vi "Intake Set Modes.vi"   [LabVIEW 2016]
uses:
  Intake Control Type.ctl
  <vilib>/Rock Robotics/WPI/DriverStation/WPI_DriverStationRobotMode2.ctl
  Intake Globals.vi
  Robot Global Data.vi
types:
  T1 = typedef "WPI_DriverStationRobotMode2.ctl" = enum16{"Autonomous Disabled", "Autonomous Enabled", "Teleop Disabled", "Teleop Enabled", "Disconnected", "Finish", "Test Disabled", "Test Enabled", "Emergency Stopped"}
  T2 = typedef "Intake Control Type.ctl" = enum16{"No Op", "In", "Out"}
  T3 = typedef "Intake Notifier.ctl" = cluster{"In":bool, "Out":bool, "Intake Control List":T2, "Parameter 1":dbl, "Parameter 2":dbl, "Intake Notifier":refnum<notifier>, "Step":i32}
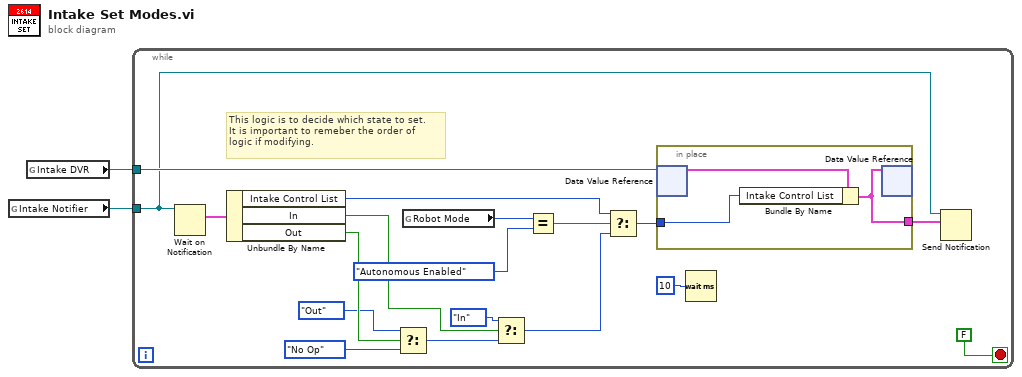
[diagram p0: block diagram]
diagram:
  n1 = global read "Intake Globals.vi" "Intake Notifier"() -> (w1:refnum<notifier>)
  n2 = global read "Intake Globals.vi" "Intake DVR"() -> (w2:refnum<data-value>)
  n3 = while {
    tunnel: w2 -> [w13]
    tunnel: w1 -> [w3]
    stop <- FALSE stop-if-true
    # "This logic is to decide which state to set. \nIt is important to remeber the order of \nlogic if modifying."
    n4 = Wait on Notification(notifier=w3) -> (notification=w18:T3)  [unwired: 3 in, 3 out]
    n5 = Unbundle By Name(w18) -> ("Intake Control List"=w4:T2, "In"=w17:bool, "Out"=w16:bool)
    n6 = Select(t=Intake_Control_Type."Out" ("Left Control List"), s=w16, f=Intake_Control_Type."No Op" ("Left Control List")) -> (s? t:f=w14:T2)
    n7 = global read "Robot Global Data.vi" "Robot Mode"() -> (w7:T1)
    n8 = Select(t=Intake_Control_Type."In" ("Intake Control List"), s=w17, f=w14) -> (s? t:f=w9:T2)
    n9 = Equal?(x=w7, y=WPI_DriverStationRobotMode2."Autonomous Enabled") -> (x = y?=w5:bool)
    n10 = Select(t=w4, s=w5, f=w9) -> (s? t:f=w8:T2)
    n11 = in-place {
      in-place-border: w8 -> [w23]
      in-place-border: [w21] -> w12
      n12 = in-place-dvr #1(w13) -> (w22:T3)  [unwired: 1 out]
      n13 = Bundle By Name(cluster=w22, "Intake Control List"=w23) -> (w21:T3)
      n14 = in-place-dvr #1(w21) -> ()  [unwired: 2 out]
    }
    n15 = Wait (ms)(milliseconds to wait=u32 10) -> ()  [unwired: 1 out]
    n16 = Send Notification(notification=w12, notifier=w3) -> ()  [unwired: 1 in, 2 out]
  }
